vi "Double2Stat.vi"(9 "error in (no error)":errorcluster, 10 "Data":dbl, 11 "Stat Address":T1 items=["Torque Enable", "Homing Complete", "Goal Id", "Goal Iq", "Goal Velo", "Goal Posi", "Present Id", "Present Iq", "Present Velo", "Present Posi", "Bus Voltage", "Temperature Winding", "Temperature MOSFET", "Temperature IC", "Error Status", "Iq_Temps"]) -> (1 "error out":errorcluster, 3 "data string":string)   [LabVIEW 2016, in "GEN_2.lvlib"]
uses:
  GEN_2.lvlib
  GEN2_Stat_Addr.ctl
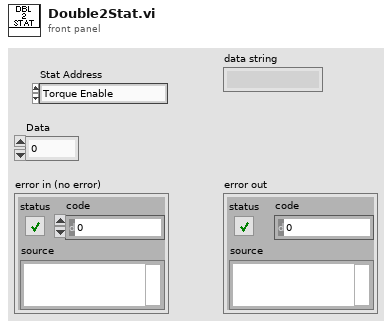
[diagram p1: front panel]
types:
  T1 = typedef "GEN_2.lvlib/GEN2_Stat_Addr.ctl" = u8
  T2 = enum16{"big-endian, network order", "native, host order", "little-endian"}
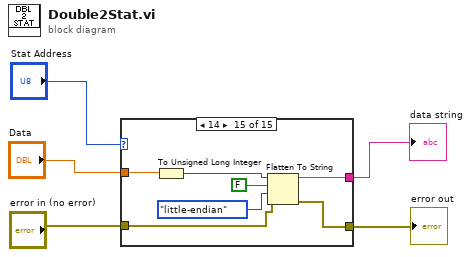
[diagram p0: block diagram]
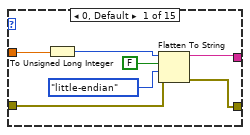
[diagram p2: hidden frame]
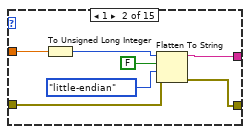
[diagram p3: hidden frame]
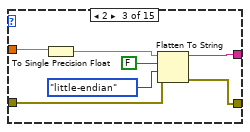
[diagram p4: hidden frame]
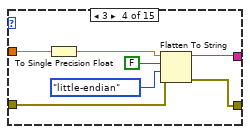
[diagram p5: hidden frame]
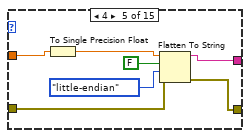
[diagram p6: hidden frame]
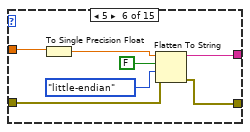
[diagram p7: hidden frame]
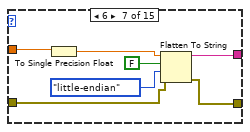
[diagram p8: hidden frame]
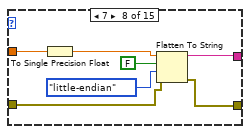
[diagram p9: hidden frame]
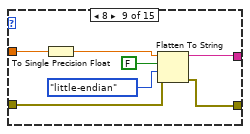
[diagram p10: hidden frame]
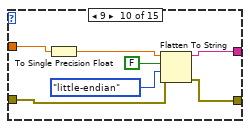
[diagram p11: hidden frame]
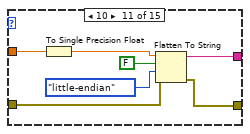
[diagram p12: hidden frame]
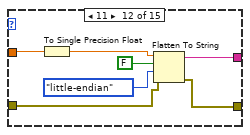
[diagram p13: hidden frame]
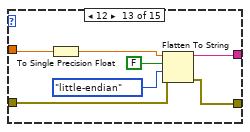
[diagram p14: hidden frame]
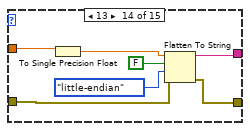
[diagram p15: hidden frame]
diagram:
  n1 = case shown="14" "Stat Address" {
    tunnel: [w9 w19 w22 w29 w36 w44 w51 w58 w62 w69 w76 w86 w90 w100 w106] -> w1
    tunnel: "Data" -> [w8 w15 w23 w30 w34 w41 w48 w55 w65 w72 w79 w83 w93 w97 w107]
    tunnel: [w6 w14 w21 w28 w37 w43 w50 w57 w63 w70 w77 w85 w91 w99 w105] -> w5
    tunnel: "error in (no error)" -> [w7 w13 w20 w27 w35 w42 w49 w56 w64 w71 w78 w84 w92 w98 w104]
    frame 0, Default {
      n2 = To Unsigned Long Integer(number=w8) -> (unsigned 32bit integer=w12:u32)
      n3 = Flatten To String(anything=w12, prepend array or string size? (T)=FALSE, byte order (0:big-endian, network order)=T2."little-endian", error in (no error)=w7) -> (data string=w9:string, error out=w6:errorcluster)  [unwired: 1 out]
    }
    frame 1 {
      n4 = To Unsigned Long Integer(number=w15) -> (unsigned 32bit integer=w16:u32)
      n5 = Flatten To String(anything=w16, prepend array or string size? (T)=FALSE, byte order (0:big-endian, network order)=T2."little-endian", error in (no error)=w13) -> (data string=w19:string, error out=w14:errorcluster)  [unwired: 1 out]
    }
    frame 2 {
      n6 = To Single Precision Float(number=w23) -> (single precision float=w24:sgl)
      n7 = Flatten To String(anything=w24, prepend array or string size? (T)=FALSE, byte order (0:big-endian, network order)=T2."little-endian", error in (no error)=w20) -> (data string=w22:string, error out=w21:errorcluster)  [unwired: 1 out]
    }
    frame 3 {
      n8 = To Single Precision Float(number=w30) -> (single precision float=w31:sgl)
      n9 = Flatten To String(anything=w31, prepend array or string size? (T)=FALSE, byte order (0:big-endian, network order)=T2."little-endian", error in (no error)=w27) -> (data string=w29:string, error out=w28:errorcluster)  [unwired: 1 out]
    }
    frame 4 {
      n10 = To Single Precision Float(number=w34) -> (single precision float=w40:sgl)
      n11 = Flatten To String(anything=w40, prepend array or string size? (T)=FALSE, byte order (0:big-endian, network order)=T2."little-endian", error in (no error)=w35) -> (data string=w36:string, error out=w37:errorcluster)  [unwired: 1 out]
    }
    frame 5 {
      n12 = To Single Precision Float(number=w41) -> (single precision float=w45:sgl)
      n13 = Flatten To String(anything=w45, prepend array or string size? (T)=FALSE, byte order (0:big-endian, network order)=T2."little-endian", error in (no error)=w42) -> (data string=w44:string, error out=w43:errorcluster)  [unwired: 1 out]
    }
    frame 6 {
      n14 = To Single Precision Float(number=w48) -> (single precision float=w52:sgl)
      n15 = Flatten To String(anything=w52, prepend array or string size? (T)=FALSE, byte order (0:big-endian, network order)=T2."little-endian", error in (no error)=w49) -> (data string=w51:string, error out=w50:errorcluster)  [unwired: 1 out]
    }
    frame 7 {
      n16 = To Single Precision Float(number=w55) -> (single precision float=w59:sgl)
      n17 = Flatten To String(anything=w59, prepend array or string size? (T)=FALSE, byte order (0:big-endian, network order)=T2."little-endian", error in (no error)=w56) -> (data string=w58:string, error out=w57:errorcluster)  [unwired: 1 out]
    }
    frame 8 {
      n18 = To Single Precision Float(number=w65) -> (single precision float=w66:sgl)
      n19 = Flatten To String(anything=w66, prepend array or string size? (T)=FALSE, byte order (0:big-endian, network order)=T2."little-endian", error in (no error)=w64) -> (data string=w62:string, error out=w63:errorcluster)  [unwired: 1 out]
    }
    frame 9 {
      n20 = To Single Precision Float(number=w72) -> (single precision float=w73:sgl)
      n21 = Flatten To String(anything=w73, prepend array or string size? (T)=FALSE, byte order (0:big-endian, network order)=T2."little-endian", error in (no error)=w71) -> (data string=w69:string, error out=w70:errorcluster)  [unwired: 1 out]
    }
    frame 10 {
      n22 = To Single Precision Float(number=w79) -> (single precision float=w80:sgl)
      n23 = Flatten To String(anything=w80, prepend array or string size? (T)=FALSE, byte order (0:big-endian, network order)=T2."little-endian", error in (no error)=w78) -> (data string=w76:string, error out=w77:errorcluster)  [unwired: 1 out]
    }
    frame 11 {
      n24 = To Single Precision Float(number=w83) -> (single precision float=w87:sgl)
      n25 = Flatten To String(anything=w87, prepend array or string size? (T)=FALSE, byte order (0:big-endian, network order)=T2."little-endian", error in (no error)=w84) -> (data string=w86:string, error out=w85:errorcluster)  [unwired: 1 out]
    }
    frame 12 {
      n26 = To Single Precision Float(number=w93) -> (single precision float=w94:sgl)
      n27 = Flatten To String(anything=w94, prepend array or string size? (T)=FALSE, byte order (0:big-endian, network order)=T2."little-endian", error in (no error)=w92) -> (data string=w90:string, error out=w91:errorcluster)  [unwired: 1 out]
    }
    frame 13 {
      n28 = To Single Precision Float(number=w97) -> (single precision float=w101:sgl)
      n29 = Flatten To String(anything=w101, prepend array or string size? (T)=FALSE, byte order (0:big-endian, network order)=T2."little-endian", error in (no error)=w98) -> (data string=w100:string, error out=w99:errorcluster)  [unwired: 1 out]
    }
    frame 14 {
      n30 = To Unsigned Long Integer(number=w107) -> (unsigned 32bit integer=w108:u32)
      n31 = Flatten To String(anything=w108, prepend array or string size? (T)=FALSE, byte order (0:big-endian, network order)=T2."little-endian", error in (no error)=w104) -> (data string=w106:string, error out=w105:errorcluster)  [unwired: 1 out]
    }
  }
  "error out" <- w5
  "data string" <- w1
